vi "why.vi"() -> ()   [LabVIEW 2023]
uses:
  Supporting VIs/Sampling frequency.ctl
  Supporting VIs/Logic states.ctl
  Supporting VIs/Motor states.ctl
  Supporting VIs/Queue names.ctl
  <instrlib>/Arcus Driver 3.0.0/ArcusUsbComm/classes/Controller/_Controller.lvclass
  <instrlib>/Arcus Driver 3.0.0/ArcusUsbComm/common/controls/linear_direction.ctl
  Supporting VIs/Axes indices.ctl
  <vilib>/DAQmx/read.llb/DAQmx Read (Analog 1D DBL NChan 1Samp).vi
  <vilib>/Analysis/baseanly.llb/Vector x A.vi
  <vilib>/Analysis/baseanly.llb/A x Vector.vi
  <vilib>/DAQmx/create/channels.llb/DAQmx Create Channel (AI-Voltage-Basic).vi
  <vilib>/DAQmx/configure/timing.llb/DAQmx Timing (Sample Clock).vi
  <vilib>/DAQmx/miscellaneous.llb/DAQmx Fill In Error Info.vi
  <vilib>/Utility/file.llb/Write Delimited Spreadsheet (string).vi
  <vilib>/Utility/file.llb/Write Delimited Spreadsheet (DBL).vi
  <vilib>/addons/control/pid/pid.llb/PID (DBL).vi
  <vilib>/Analysis/NI_AALBase.lvlib
  <instrlib>/Arcus Driver 3.0.0/ArcusUsbComm/libraries/common.lvlib
  <vilib>/addons/control/pid/NI_PID_pid.lvlib
  <instrlib>/Zaber A Series/Zaber A Series.lvlib
panel:
  out "Steady State COFs":dbl[](array[numeric])
  out "Fixed amplitude Load":dbl(graph)=8.923720573303449
  in  "VISA resource name":refnum<visa-resource-name>
  out "Mean Estimated Friction Coefficient":dbl[](array[numeric])
  in  "Maximum COF Difference":i32=3000
  in  "Number of Previous Points":i32=3000
  out "Torque":dbl(graph)=-1.1532615270996815
  out "Sliding Distance (mm)":i32
  out "Angular Position":dbl
  in  "Initial Position":dbl
  in  "Track Radius (mm)":T1=100 items=["4 mm"=4, "6 mm"=6, "8 mm"=8, "10 mm"=10, "12 mm"=12, "14 mm"=14, "16 mm"=16, "18 mm"=18]
  out "Revolutions Completed":u8(slide) scale=0.0..10.0
  in  "STOP Rotating Motor":bool
  in  "Clockwise":bool
  in  "Number of Revolutions":i32
  out "Progress":dbl(slide) scale=0.0..100.0
  in  "Velocity":dbl
  in  "Units (0: microsteps)":u16(ring) items=["device speed units", "microns per second", "millimeters per second", "inches per second", "degrees per second"]
  in  "Microstep Size (0)":dbl
  in  "Wait [min]":dbl=30.0 format="%.2g"
  in  "Wait ?":bool=TRUE
  in  "Save file name":path=path "C:/Users/Egberts/Desktop/Tribometer/August 2020 Measurements/Tribometer/Late August 2020/test.txt"
  in  "PID gains":T2={"proportional gain (Kc)"=0.02, "integral time (Ti, min)"=0.1, "derivative time (Td, min)"=0.001} {"derivative time (Td, min)" format="%.3f"; "integral time (Ti, min)" format="%.3f"; "proportional gain (Kc)" format="%.3f"}
  in  "output range":cluster{"output high":dbl, "output low":dbl}={"output high"=2.0, "output low"=-2.0} {"output low" format="%.2f"; "output high" format="%.2f"}
  out "x-position":i32
  out "z-position":string
  in  "set zero":bool
  out "Correction loop":i32
  out "received P":i32
  out "Actual Load":dbl
  out "Correction [N]":dbl format="%.2f"
  out "correction [p]":dbl
  out "to PID":i32
  out "dt out (s)":dbl=0.25 format="%.3f"
  in  "Testing Load [N]":dbl=20.0
  in  "Wear cycles":i32=3000
  out "Manual control":bool
  in  "Approach":bool
  in  "DAQmx Device Name":tag="Dev1"
  in  "Out":bool
  in  "In":bool
  in  "Left":bool
  in  "Right":bool
  in  "Up":bool
  out "Estimated friction coefficient":dbl(graph)=-0.11599973982411911
  out "Smooth Force from Torque":dbl(graph)=-1.1532615270996815
  out "Smooth z":dbl(graph)=9.94193201509139
  out "Dequeued Data":dbl[](graph)=[9.378691263157721, 10.717600289594278, 8.438969804942502, 9.318124790458075, 8.681089909963866, 9.970529667476073, 10.834102440336615, 9.183821958337319, 9.334582664259113, 9.226213467034226, 10.238553338370796, 11.173780758664948, 8.690449558950064, 9.261606371512476, 8.790570665988898, 9.887706352746802, 11.038667014275244, 8.916330650848511, 9.104119720861869, 8.923720573303449]
  in  "ABORT":bool
  in  "Down":bool
  out "Aborted":bool
  out "Mean z":dbl[](array[numeric])
  out "Current reading":dbl[](array[numeric])
  in  "Averaging Level":i32=12
  out "Mean Force from Torque":dbl[](array[numeric])
  out "Completed":bool
  out "Testing":bool
  out "Approaching":bool
  in  "TARE":bool
  in  "Sampling frequency (rate)":T1=100 items=["1000 Hz"=1000, " 500 Hz"=500, " 250 Hz"=250, "100 Hz"=100, "50 Hz"=50, "10 Hz"=10, "1 Hz"=1]
  in  "Calibration file":path=path "C:/Users/Egberts/Desktop/ATI Industrial Automation/FT21774.cal"
  # "Counterclockwise"
  # "Originally used to measure \nthe amount of positions needed\nto perform fast approach"
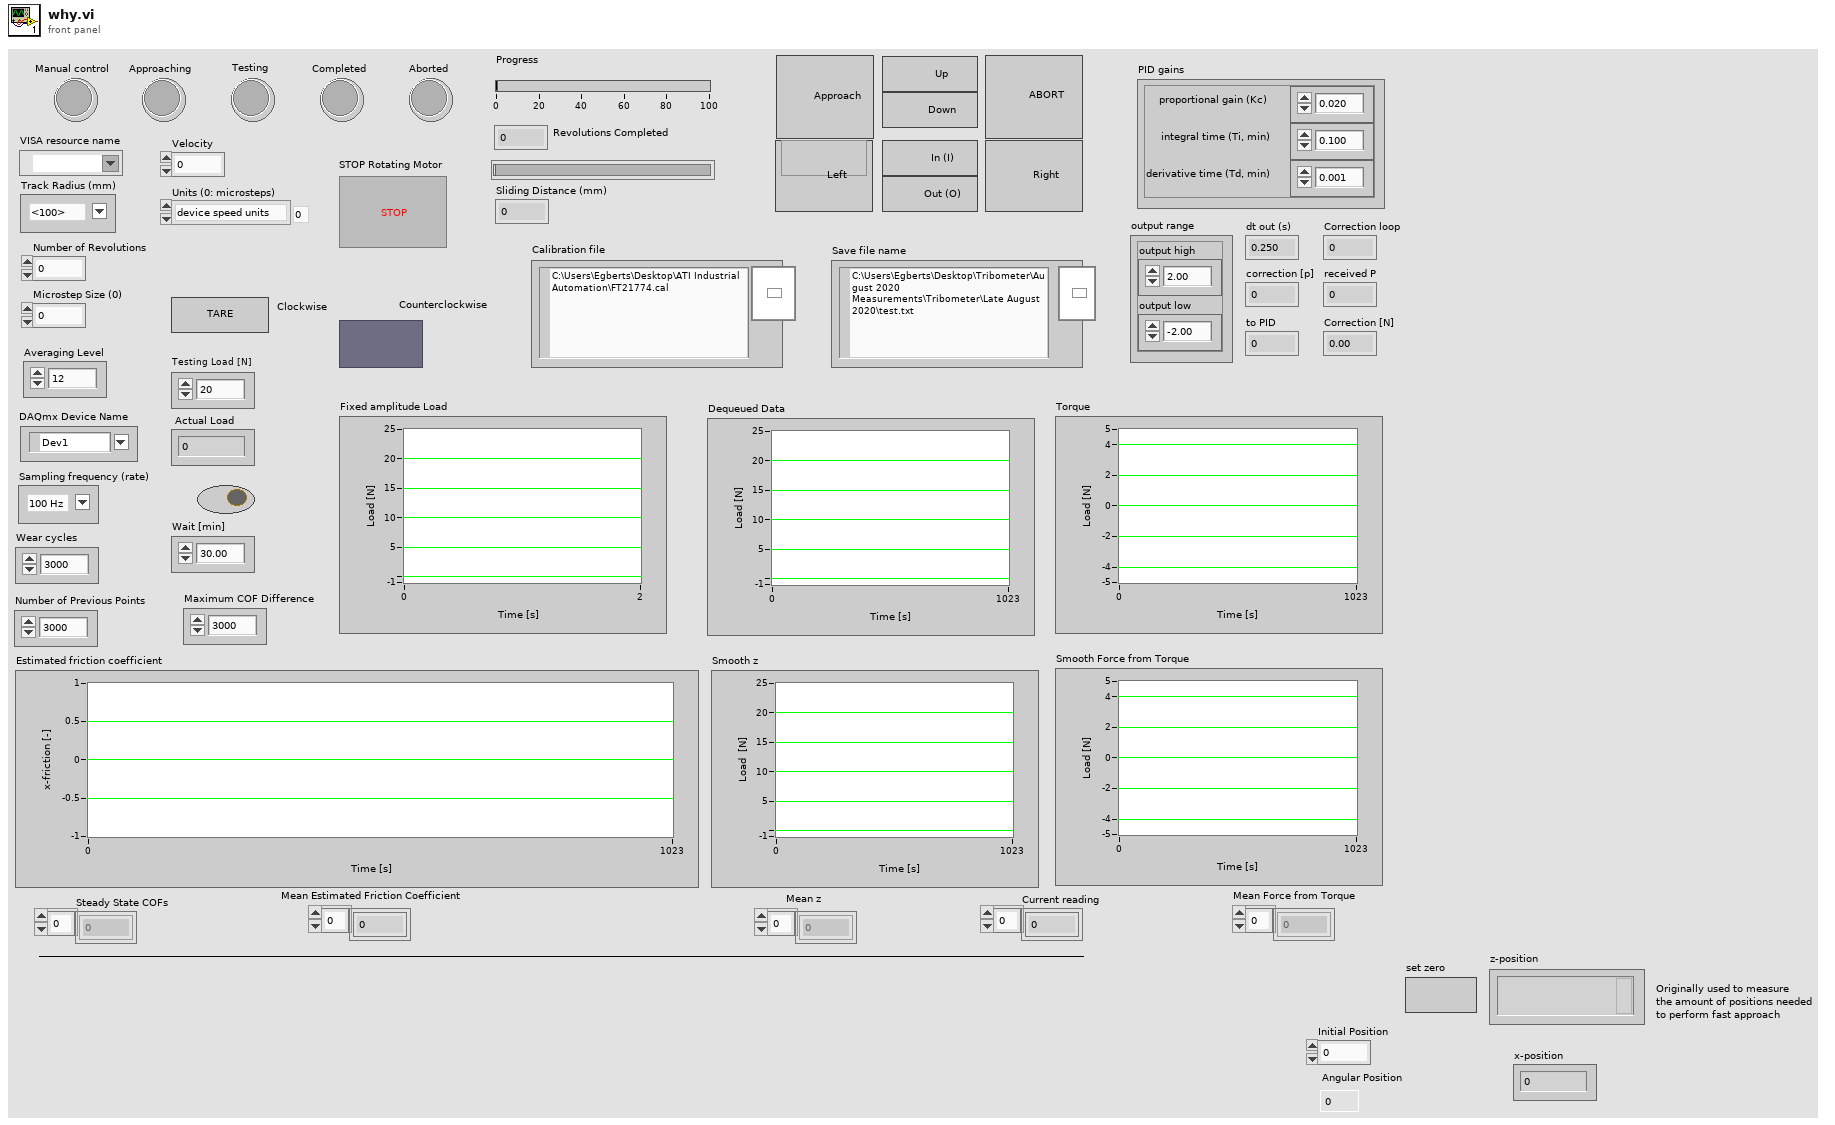
[diagram p1: front panel]
types:
  T1 = typedef "Sampling frequency.ctl" = u16
  T2 = cluster{"proportional gain (Kc)":dbl, "integral time (Ti, min)":dbl, "derivative time (Td, min)":dbl}
  T3 = typedef "Queue names.ctl" = enum16{"Cell queue name", "z-axis ref queue", "x-axis ref queue", "tangent-axis ref queue", "y-axis ref queue", "to PID", "Feedback"}
  T4 = typedef "Motor states.ctl" = enum16{"Initialize", "Manual control", "Approaching", "Testing", "Terminate"}
  T5 = typedef "Logic states.ctl" = enum16{"Initialize", "Process", "Terminate"}
  T6 = enum8{"Enabled", "Disabled", "Disabled and Grayed Out"}
  T7 = cluster{"queue out":refnum<queue>, "error out":errorcluster}
  T8 = cluster{"task out":refnum<k21>, "error out":errorcluster}
  T9 = cluster{"reference (out)":refnum<class "_Controller.lvclass">, "error out":errorcluster}
  T10 = typedef "Axes indices.ctl" = enum16{"y-axis", "x-axis", "z-axis"}
  T11 = cluster{"queue out":refnum<queue>, "queue out":refnum<queue>, "queue out":refnum<queue>}
  T12 = typedef "common.lvlib/linear_direction.ctl" = enum16{"POS (+)", "NEG (-)"}
  T13 = typedef "lveventtype.ctl" = enum32{"Null", "Timeout", "Annotation Menu Selection", "Annotation Menu Selection?", "App Instance Close", "App Instance Close?", "Autoscale Range Change", "Bookmark Info Change", "Cell Edit", "Cell Edit?", "Cursor Grab", "Cursor Grab?", "Cursor Menu Selection", "Cursor Menu Selection?", "Cursor Move", "Cursor Release", "Data Change", "Direction Change", "Display State Change", "Drag Ended", "Drag Enter", "Drag Leave", "Drag Over", "Drag Source Update", "Drag Starting", "Drag Starting?", "Drop", "Exec State Change", "Key Down", "Key Down?", "Key Repeat", "Key Repeat?", "Key Up", "Listbox Double Click", "Menu Activation?", "Menu Selection (App)", "Menu Selection? (App)", "Menu Selection (User)", "Mouse Down", "Mouse Down?", "Mouse Enter", "Mouse Leave", "Mouse Move", "Mouse Up", "Mouse Wheel", "NI Security User Change (App)", "Pane Size", "Panel Close", "Panel Close?", "Panel Resize", "Plot Attribute Change", "Scale Range Change", "Shortcut Menu Activation?", "Shortcut Menu Selection (App)", "Shortcut Menu Selection? (App)", "Shortcut Menu Selection (User)", "Tree Double Click", "Tree Drag", "Tree Drag?", "Tree Drop", "Tree Drop?", "Tree Item Close", "Tree Item Close?", "Tree Item Open", "Tree Item Open?", "User Event", "Value Change"}
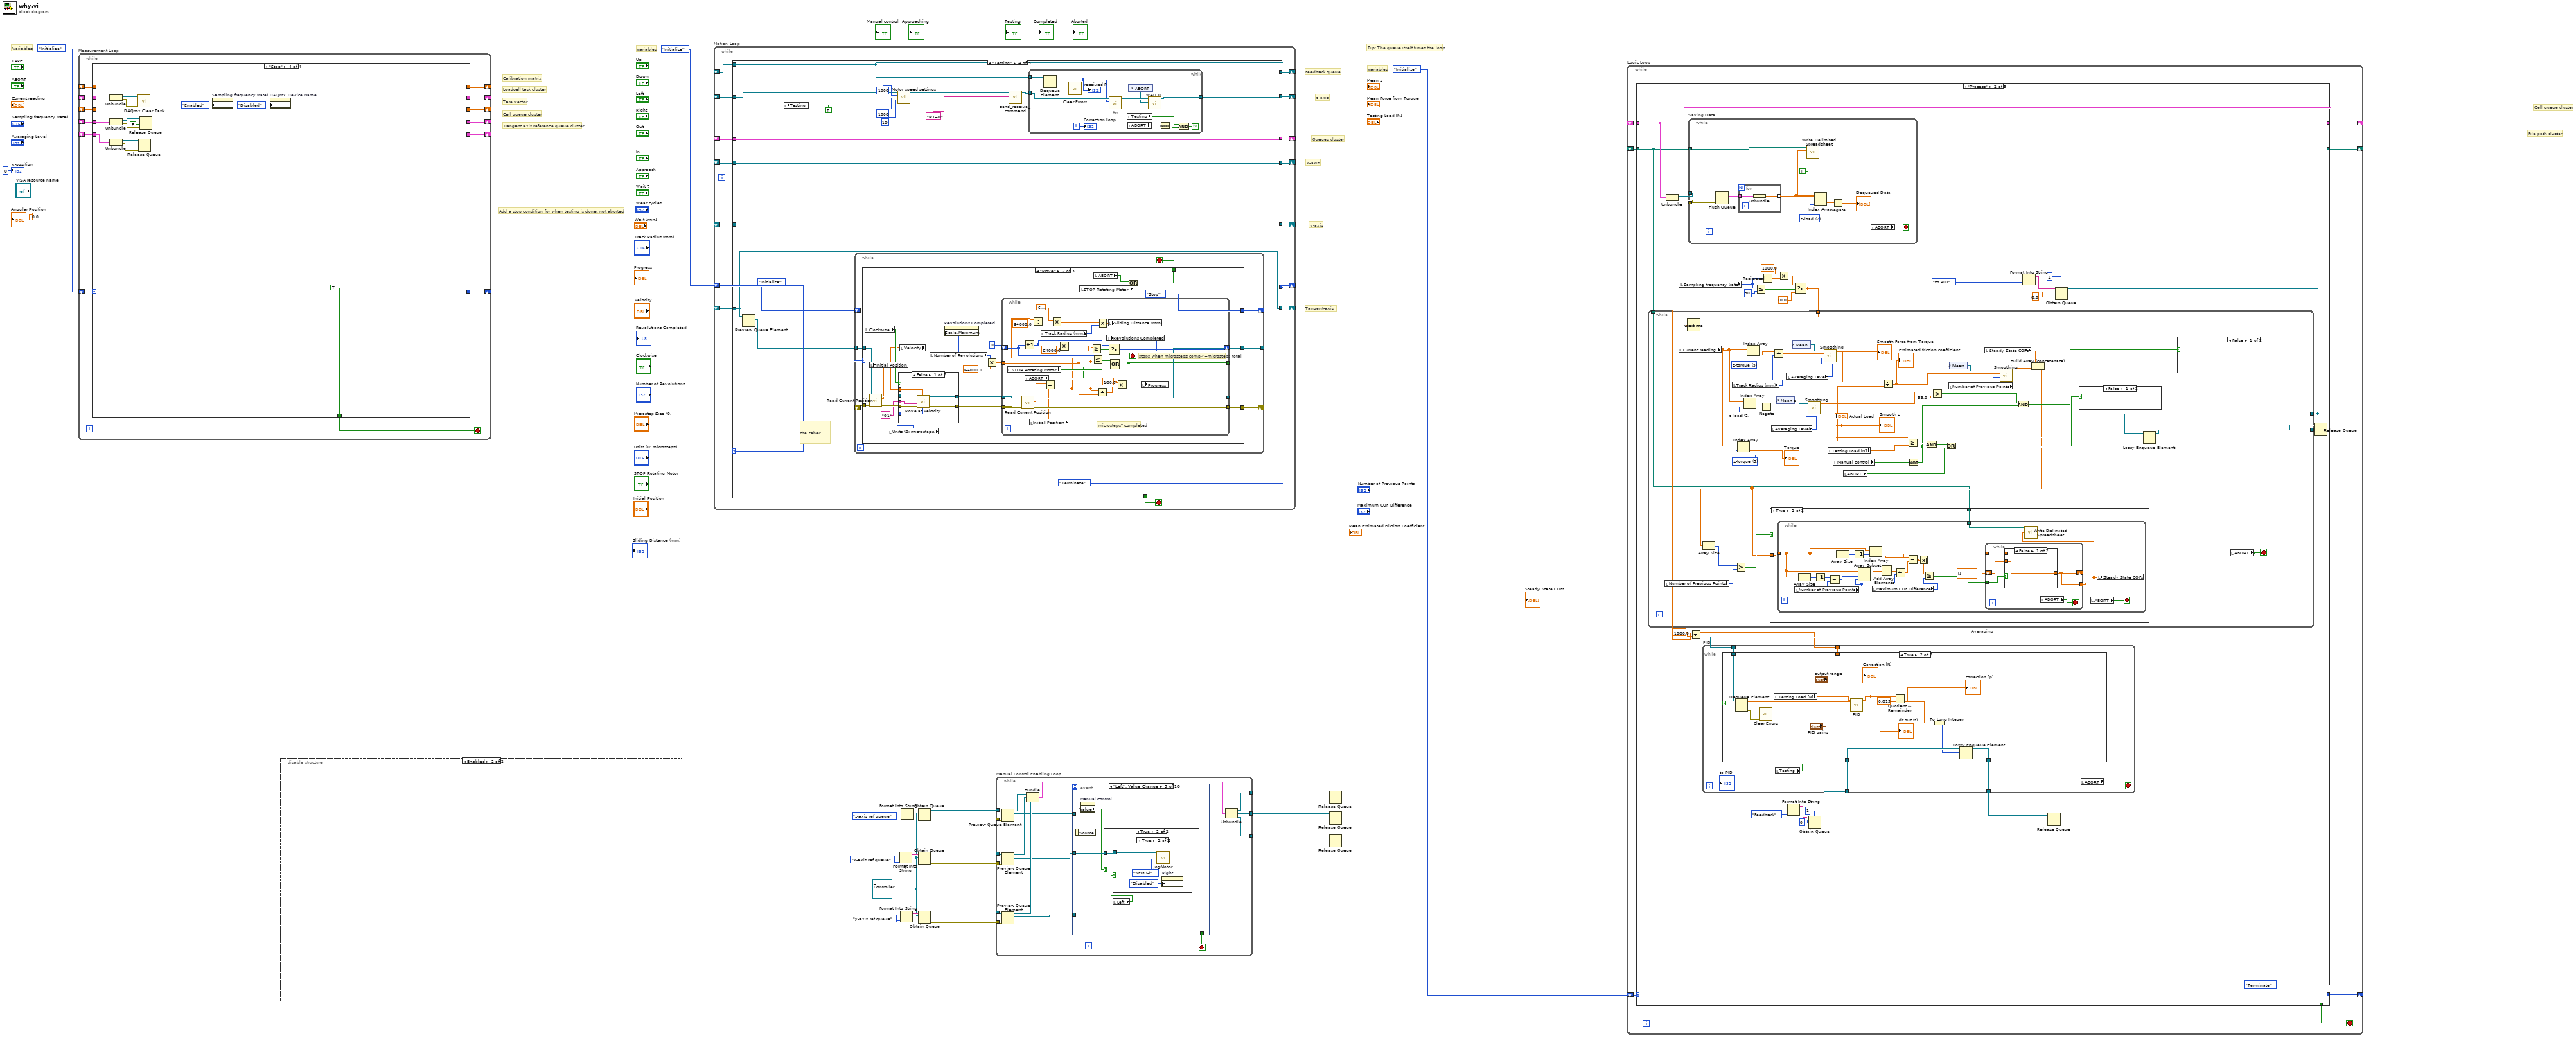
[diagram p0: block diagram]
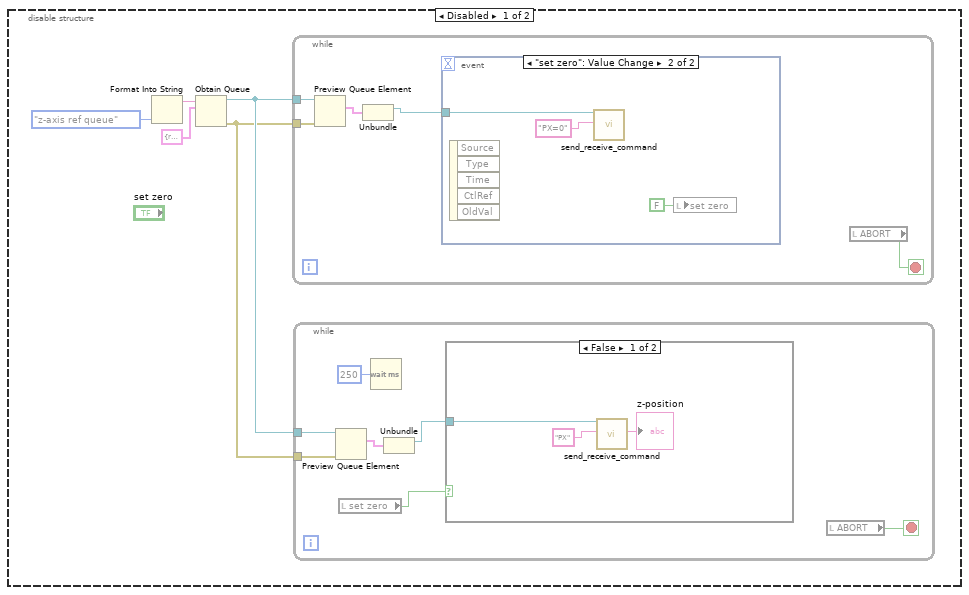
[diagram p2: hidden frame]
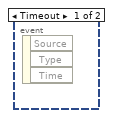
[diagram p4: hidden frame]
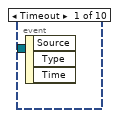
[diagram p5: hidden frame]
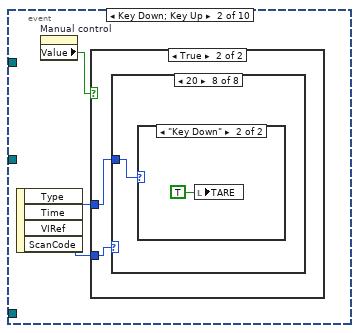
[diagram p6: hidden frame]
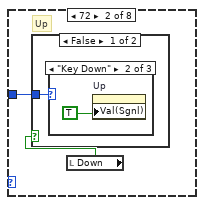
[diagram p9: hidden frame]
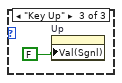
[diagram p11: hidden frame]
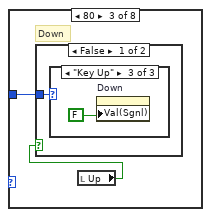
[diagram p13: hidden frame]
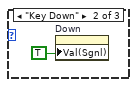
[diagram p15: hidden frame]
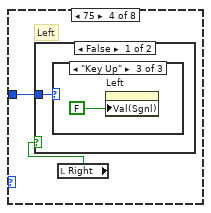
[diagram p17: hidden frame]
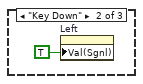
[diagram p19: hidden frame]
diagram:
  w2 = refnum<class "_Controller.lvclass"> refnum ("Controller in")
  # "Tangent-axis"
  # "Feedback queue"
  # "Queues cluster"
  # "Tangent axis reference queue cluster"
  # "Add a stop condition for when testing is done, not aborted"
  # "y-axis"
  # "x-axis"
  # "z-axis"
  # "Variables"
  # "Variables"
  # "File path cluster"
  # "Cell queue cluster"
  # "Tip: The queue itself times the loop"
  # "Variables"
  # "Cell queue cluster"
  # "Loadcell task cluster"
  # "Tare vector"
  # "Calibration matrix"
  n1 = while "Measurement Loop" {
    shift-right: [w33] -> _
    shift-left: enum16{"Initialize", "Tare", "Measure", "Stop"}."Initialize" ("Enum") -> [w34]
    shift-right: [w28] -> _
    shift-left: _ -> [w27]
    shift-right: [w32] -> _
    shift-left: _ -> [w30]
    shift-right: [w31] -> _
    shift-left: _ -> [w29]
    shift-right: [w24] -> _
    shift-left: _ -> [w25]
    shift-right: [w23] -> _
    shift-left: _ -> [w22]
    stop <- w26 stop-if-true
    n2 = case shown="\"Stop\"" w34 {
      tunnel: [w57 w82 w117 _] -> w33
      tunnel: [_ w89 _ _] -> w32
      tunnel: [w61 w81 w119 _] -> w31
      tunnel: w29 -> [_ w81 w119 w185]
      tunnel: w30 -> [_ _ w120 _]
      tunnel: [w60 w88 w118 _] -> w28
      tunnel: w27 -> [_ w88 w118 _]
      tunnel: [_ _ _ TRUE] -> w26
      tunnel: w25 -> [_ w76 w105 w182]
      tunnel: [w52 w76 w106 _] -> w24
      tunnel: [w41 w74 w113 _] -> w23
      tunnel: w22 -> [_ w74 w113 w176]
      frame "Initialize", Default {
        w65 = u16 10123 items=["Continous"=10123, "Finite"=10178, "Hardware Timed"=12522]  # Sample mode
        w72 = "N-M"  # Torque units
        w71 = "N"  # Force units
        n3 = local read "VISA resource name"() -> (w36:refnum<visa-resource-name>)
        n4 = property on="Sampling frequency (rate)" class="Ring (strict)"("DisabledEnum"=T6."Disabled" ("Disabled")) -> ()  [unwired: 2 in, 2 out]
        n5 = call "mxChannelList.vi"("First Channel"=0, "Number of Channels"=6, "DAQmx Device Name"="DAQmx Device Name") -> ("error out"=w67:errorcluster, "Channel List"=w68:string)  [unwired: 1 in]
        n6 = call <instrlib>:"Initialize.vi"("VISA resource name"=w36) -> ("VISA resource name out"=w35:refnum<visa-resource-name>)  [unwired: 9 in, 1 out]
        n7 = call "LoadCalibrationFromFile.vi"("User Torque Units"=w72, "User Force Units"=w71, "Cal File Path"="Calibration file") -> ("Calibration Matrix"=w60:dbl[][])  [unwired: 1 in, 3 out]
        n8 = property on="DAQmx Device Name" class="DAQmxName"("DisabledEnum"=T6."Disabled" ("Disabled")) -> ()  [unwired: 2 in, 2 out]
        n9 = Format Into String(Queue_names."Cell queue name" ("Enum")) -> (resulting string=w39:string)  [unwired: 3 in, 1 out]
        n10 = call-poly <vilib>:"DAQmx Create Virtual Channel.vi"("physical channels"=w68, "error in"=w67) -> ("task out"=w66:refnum<k21>, "error out"=w45:errorcluster)  [unwired: 12 in]
        n11 = local read "Sampling frequency (rate)"() -> (w51:T1)
        n12 = call-poly <vilib>:"DAQmx Timing.vi"("task/channels in"=w66, "sample mode"=w65, "rate"=w51) -> ("task out"=w64:refnum<k21>, "error out"=w63:errorcluster)  [unwired: 11 in]
        n13 = Format Into String(Queue_names."tangent-axis ref queue" ("Enum")) -> (resulting string=w37:string)  [unwired: 3 in, 1 out]
        n14 = call <vilib>:"DAQmx Start Task.vi"("task/channels in"=w64, "error in"=w63) -> ("task out"=w62:refnum<k21>, "error out"=w46:errorcluster)  [unwired: 12 in]
        n15 = Obtain Queue(name (unnamed)=w37, element data type=w35) -> (queue out=w43:refnum<queue>, error out=w42:errorcluster)  [unwired: 3 in, 1 out]
        n16 = Obtain Queue(name (unnamed)=w39, element data type=dbl[] []) -> (queue out=w53:refnum<queue>, error out=w47:errorcluster)  [unwired: 3 in, 1 out]
        n17 = local read "ABORT"() -> (w55:bool)
        n18 = Bundle("queue out"=w53, "error out"=w47) -> (w52:T7)  [unwired: 1 in]
        n19 = Bundle("queue out"=w43, "error out"=w42) -> (w41:T7)  [unwired: 1 in]
        n20 = Bundle("task out"=w62, "error out"=w46) -> (w61:T8)  [unwired: 1 in]
        n21 = Merge Errors(w42, w47, w46, w45) -> (w44:errorcluster)
        n22 = Compound Arithmetic op=OR(w44, w55) -> (w56:bool)
        n23 = Select(t=enum16{"Initialize", "Tare", "Measure", "Stop"}."Stop" ("Enum"), s=w56, f=enum16{"Initialize", "Tare", "Measure", "Stop"}."Tare" ("Enum")) -> (s? t:f=w57:enum16{"Initialize", "Tare", "Measure", "Stop"})
      }
      frame "Tare" {
        n24 = local read "Averaging Level"() -> (w75:i32)
        n25 = for {
          N: w75 -> [_]
          tunnel: w81 -> [w95]
          shift-right: [w97] -> w79
          shift-left: dbl[][] [] -> [w96]
          tunnel: [w94] -> w78
          tunnel: [FALSE] -> w77
          n26 = Unbundle(w95) -> ("task out"=w100:refnum<k21>, "error out"=w99:errorcluster)
          n27 = call-poly <vilib>:"DAQmx Read.vi"("task/channels in"=w100, "error in"=w99) -> ("data"=w98:dbl[], "error out"=w94:errorcluster)  [unwired: 11 in, 1 out]
          n28 = Build Array (concatenate)(w96, w98) -> (w97:dbl[][])
        }
        n29 = local write "TARE"(w77) -> ()
        n30 = Matrix Size(0:w79) -> (1:w90:i32)  [unwired: 1 out]
        n31 = Reciprocal(x=w90) -> (1/x=w91:dbl)
        n32 = Unbundle By Name(w78) -> ("status"=w83:bool)
        n33 = local read "ABORT"() -> (w84:bool)
        n34 = Initialize Array(w91, w90) -> (w92:dbl[])
        n35 = Or(x=w83, y=w84) -> (x .or. y?=w87:bool)
        n36 = call-poly <vilib>:"A x B.vi"("Matrix A"=w79, "Vector V'"=w92) -> ("V' x A"=w89:dbl[])  [unwired: 1 out]
        n37 = Select(t=enum16{"Initialize", "Tare", "Measure", "Stop"}."Stop" ("Enum"), s=w87, f=enum16{"Initialize", "Tare", "Measure", "Stop"}."Measure" ("Enum")) -> (s? t:f=w82:enum16{"Initialize", "Tare", "Measure", "Stop"})
      }
      frame "Measure" {
        n38 = Unbundle(w113) -> ("queue out"=w102:refnum<queue>, "error out"=w101:errorcluster)
        n39 = Unbundle(w105) -> ("queue out"=w104:refnum<queue>, "error out"=w103:errorcluster)
        n40 = Unbundle(w113) -> ("queue out"=w112:refnum<queue>, "error out"=w111:errorcluster)
        n41 = Unbundle(w119) -> ("task out"=w110:refnum<k21>, "error out"=w109:errorcluster)
        n42 = while {
          tunnel: w120 -> [w161]
          tunnel: w118 -> [w153]
          tunnel: [w151] -> w114
          tunnel: w112 -> [w144]
          tunnel: w111 -> [w143]
          tunnel: w110 -> [w142]
          tunnel: w109 -> [w141]
          tunnel: [w140] -> w108
          tunnel: [w139] -> w107
          tunnel: w104 -> [w138]
          tunnel: w103 -> [w137]
          stop <- w156 stop-if-true
          w158 = u16 2 items=["x-load", "y-load", "z-load", "x-torque", "y-torque", "z-torque"]
          n43 = Get Queue Status(queue=w144, error in (no error)=w143) -> (# elements in queue=w148:i32)  [unwired: 1 in, 7 out]
          n44 = local read "Testing"() -> (w147:bool)
          n45 = call-poly <vilib>:"DAQmx Read.vi"("task/channels in"=w142, "error in"=w141) -> ("data"=w154:dbl[], "error out"=w152:errorcluster)  [unwired: 11 in, 1 out]
          n46 = Not Equal To 0?(x=w148) -> (x != 0?=w146:bool)
          n47 = And(x=w146, y=w147) -> (x .and. y?=w145:bool)
          n48 = Subtract(x=w154, y=w161) -> (x-y=w160:dbl[])
          n49 = call-poly <vilib>:"A x B.vi"("Vector"=w160, "A"=w153) -> ("A x Vector"=w149:dbl[])  [unwired: 1 out]
          n50 = case shown="True" w145 {
            tunnel: [FALSE ("status") w173] -> w150
            tunnel: w149 -> [_ w172]
            tunnel: w138 -> [w163 w170]
            tunnel: w137 -> [w162 w169]
            tunnel: [w163 w168] -> w140
            tunnel: [w162 w167] -> w139
            frame False {
            }
            frame True {
              n51 = local read "Angular Position"() -> (w165:dbl)
              n52 = To Long Integer(number=w165) -> (32bit integer=w166:i32)
              n53 = Build Array (concatenate)(w172, w166) -> (w171:dbl[])
              n54 = Enqueue Element(queue=w170, element=w171, error in (no error)=w169) -> (queue out=w168:refnum<queue>, error out=w167:errorcluster)  [unwired: 1 in, 1 out]
              n55 = Unbundle By Name(w167) -> ("status"=w173:bool)
            }
          }
          n56 = local write "Current reading"(w149) -> ()
          n57 = Index Array(array=w149, index=w158) -> (element=w159:dbl)
          n58 = Negate(x=w159) -> (-x=→"Fixed amplitude Load":dbl)
          n59 = local read "TARE"() -> (w151:bool)
          n60 = Unbundle By Name(w152) -> ("status"=w155:bool)
          n61 = local read "ABORT"() -> (w157:bool)
          n62 = Compound Arithmetic op=OR(w150, w151, w157, w155) -> (w156:bool)
        }
        n63 = while {
          tunnel: w102 -> [w122]
          tunnel: w101 -> [w121]
          stop <- w124 stop-if-true
          n64 = local read "Testing"() -> (w128:bool)
          n65 = Get Queue Status(queue=w122, error in (no error)=w121) -> (queue out=w126:refnum<queue>, # elements in queue=w130:i32)  [unwired: 1 in, 6 out]
          n66 = Not Equal To 0?(x=w130) -> (x != 0?=w129:bool)
          n67 = And(x=w129, y=w128) -> (x .and. y?=w127:bool)
          n68 = case shown="True" w127 {
            tunnel: w126 -> [_ w134]
            frame False {
            }
            frame True {
              n69 = Preview Queue Element(queue=w134) -> (element=w133:refnum<visa-resource-name>)  [unwired: 2 in, 3 out]
              n70 = call <instrlib>:"Read Current Position.vi"("Device and Axis"="PX", "VISA resource name"=w133) -> ("VISA resource name out"=w131:refnum<visa-resource-name>)  [unwired: 7 in, 2 out]
              n71 = Decimal String To Number(string=w131) -> (number=w135:i32)  [unwired: 2 in, 1 out]
              n72 = local write "Angular Position"(w135) -> ()
            }
          }
          n73 = local read "ABORT"() -> (w125:bool)
          n74 = local read "TARE"() -> (w123:bool)
          n75 = Or(x=w125, y=w123) -> (x .or. y?=w124:bool)
        }
        n76 = Select(t=enum16{"Initialize", "Tare", "Measure", "Stop"}."Tare" ("Enum"), s=w114, f=enum16{"Initialize", "Tare", "Measure", "Stop"}."Stop" ("Enum")) -> (s? t:f=w117:enum16{"Initialize", "Tare", "Measure", "Stop"})
        n77 = Bundle("queue out"=w108, "error out"=w107) -> (w106:T7)  [unwired: 1 in]
      }
      frame "Stop" {
        n78 = Unbundle(w185) -> ("task out"=w184:refnum<k21>, "error out"=w183:errorcluster)
        n79 = Unbundle(w182) -> ("queue out"=w181:refnum<queue>, "error out"=w180:errorcluster)
        n80 = Unbundle(w176) -> ("queue out"=w175:refnum<queue>, "error out"=w174:errorcluster)
        n81 = call <vilib>:"DAQmx Clear Task.vi"("task in"=w184, "error in"=w183) -> ()  [unwired: 13 in, 1 out]
        n82 = Release Queue(queue=w175, error in (no error)=w174) -> ()  [unwired: 1 in, 3 out]
        n83 = Release Queue(queue=w181, force destroy? (F)=FALSE, error in (no error)=w180) -> ()  [unwired: 3 out]
        n84 = property on="Sampling frequency (rate)" class="Ring (strict)"("DisabledEnum"=T6."Enabled" ("Disabled")) -> ()  [unwired: 2 in, 2 out]
        n85 = property on="DAQmx Device Name" class="DAQmxName"("DisabledEnum"=T6."Disabled" ("Disabled")) -> ()  [unwired: 2 in, 2 out]
      }
    }
  }
  n86 = disable-structure shown="Enabled" {
    frame Disabled {
      n87 = Format Into String(Queue_names."z-axis ref queue" ("Enum")) -> (resulting string=w190:string)  [unwired: 3 in, 1 out]
      n88 = Obtain Queue(name (unnamed)=w190, element data type=T9 {"reference (out)"=refnum, "error out"={"status"=FALSE, "code"=0, "source"=""}} ("output cluster")) -> (queue out=w188:refnum<queue>, error out=w187:errorcluster)  [unwired: 3 in, 1 out]
      n89 = while {
        tunnel: w188 -> [w206]
        tunnel: w187 -> [w205]
        stop <- w202 stop-if-true
        n90 = Preview Queue Element(queue=w206, error in (no error)=w205) -> (element=w204:T9)  [unwired: 1 in, 3 out]
        n91 = Unbundle(w204) -> ("reference (out)"=w203:refnum<class "_Controller.lvclass">)  [unwired: 1 out]
        n92 = event shown="[1] \"set zero\": Value Change" {
          selector: _ -> [_ _]
          dyn-events: _ -> [_ _]
          timeout: _ -> [_ _]
          tunnel: w203 -> [_ w209]
          event Timeout {
            n93 = event-data() -> ()  [unwired: 1 in, 3 out]
          }
          event "set zero": Value Change {
            n94 = event-data() -> ()  [unwired: 1 in, 5 out]
            n95 = call <instrlib>:"send_receive_command.vi"("reference (in)"=w209, "ASCII Command (in)"="PX=0") -> ()  [unwired: 13 in, 5 out]
            n96 = local write "set zero"(FALSE ("set zero")) -> ()
          }
        }
        n97 = local read "ABORT"() -> (w202:bool)
      }
      n98 = while {
        tunnel: w188 -> [w195]
        tunnel: w187 -> [w194]
        stop <- w197 stop-if-true
        n99 = Preview Queue Element(queue=w195, error in (no error)=w194) -> (element=w196:T9)  [unwired: 1 in, 3 out]
        n100 = local read "set zero"() -> (w192:bool)
        n101 = Wait (ms)(milliseconds to wait=u32 250) -> ()  [unwired: 1 out]
        n102 = Unbundle(w196) -> ("reference (out)"=w193:refnum<class "_Controller.lvclass">)  [unwired: 1 out]
        n103 = case shown="False" w192 {
          tunnel: w193 -> [w200 _]
          frame False {
            n104 = call <instrlib>:"send_receive_command.vi"("reference (in)"=w200, "ASCII Command (in)"="PX") -> ("response (out)"=→"z-position":string)  [unwired: 13 in, 4 out]
          }
          frame True {
          }
        }
        n105 = local read "ABORT"() -> (w197:bool)
      }
    }
    frame Enabled {
    }
  }
  n106 = while "Motion Loop" {
    shift-right: [w223] -> _
    shift-left: Motor_states."Initialize" -> [w224]
    shift-right: [w215] -> _
    shift-left: _ -> [w222]
    shift-right: [w214] -> _
    shift-left: _ -> [w212]
    shift-right: [w213] -> _
    shift-left: _ -> [w221]
    shift-right: [w219] -> _
    shift-left: _ -> [w218]
    shift-right: [w217] -> _
    shift-left: _ -> [w216]
    shift-right: [w211] -> _
    shift-left: _ -> [w210]
    stop <- w220 stop-if-true
    n107 = case shown="\"Testing\"" w224 {
      tunnel: [Motor_states."Manual control" w294 w316 Motor_states."Terminate" _] -> w223
      tunnel: w222 -> [_ w279 w307 w365 w478]
      tunnel: w221 -> [_ w275 w309 w363 w476]
      tunnel: [_ _ _ _ w484] -> w220
      tunnel: [w243 w281 w312 w370 _] -> w219
      tunnel: w218 -> [_ w281 w312 w370 w483]
      tunnel: [w238 w280 w311 w369 _] -> w217
      tunnel: w216 -> [_ w280 w311 w369 w479]
      tunnel: [w237 w278 w310 w364 _] -> w215
      tunnel: [w236 w276 w304 w362 _] -> w214
      tunnel: [w235 w274 w309 w363 _] -> w213
      tunnel: w212 -> [_ w277 w305 w362 w477]
      tunnel: [w228 w273 w303 w359 _] -> w211
      tunnel: w210 -> [_ w273 w303 w359 _]
      frame "Initialize" {
        w225 = TRUE
        w234 = FALSE ("Approach")
        n108 = local write "Testing"(w234) -> ()
        n109 = local write "Aborted"(w234) -> ()
        n110 = local write "Approach"(w234) -> ()
        n111 = local write "Approaching"(w234) -> ()
        n112 = local write "Completed"(w234) -> ()
        n113 = local write "Progress"(0 ("Test Progress")) -> ()
        n114 = local read "VISA resource name"() -> (w230:refnum<visa-resource-name>)
        n115 = call <instrlib>:"initialize.vi"("device_index (in) [0=def]"=Axes_indices."x-axis", "clear_buffer? (T)"=w225) -> ("reference (out)"=w267:refnum<class "_Controller.lvclass">)  [unwired: 16 in, 1 out]
        n116 = call <instrlib>:"initialize.vi"("device_index (in) [0=def]"=Axes_indices."y-axis", "clear_buffer? (T)"=w225) -> ("reference (out)"=w266:refnum<class "_Controller.lvclass">)  [unwired: 16 in, 1 out]
        n117 = call <instrlib>:"initialize.vi"("device_index (in) [0=def]"=Axes_indices."z-axis", "clear_buffer? (T)"=w225) -> ("reference (out)"=w268:refnum<class "_Controller.lvclass">)  [unwired: 16 in, 1 out]
        n118 = call <instrlib>:"send_receive_command.vi"("reference (in)"=w267, "ASCII Command (in)"="SR0=0") -> ("reference (out)"=w261:refnum<class "_Controller.lvclass">)  [unwired: 13 in, 4 out]
        n119 = call <instrlib>:"send_receive_command.vi"("reference (in)"=w266, "ASCII Command (in)"="SR0=0") -> ("reference (out)"=w262:refnum<class "_Controller.lvclass">)  [unwired: 13 in, 4 out]
        n120 = call <instrlib>:"send_receive_command.vi"("reference (in)"=w268, "ASCII Command (in)"="SR0=0") -> ("reference (out)"=w260:refnum<class "_Controller.lvclass">)  [unwired: 13 in, 4 out]
        n121 = call <instrlib>:"Initialize.vi"("VISA resource name"=w230) -> ("VISA resource name out"=w226:refnum<visa-resource-name>)  [unwired: 9 in, 1 out]
        n122 = call <instrlib>:"send_receive_command.vi"("reference (in)"=w261, "ASCII Command (in)"="INC") -> ("reference (out)"=w236:refnum<class "_Controller.lvclass">)  [unwired: 13 in, 4 out]
        n123 = call <instrlib>:"send_receive_command.vi"("reference (in)"=w262, "ASCII Command (in)"="INC") -> ("reference (out)"=w235:refnum<class "_Controller.lvclass">)  [unwired: 13 in, 4 out]
        n124 = call <instrlib>:"send_receive_command.vi"("reference (in)"=w260, "ASCII Command (in)"="INC") -> ("reference (out)"=w237:refnum<class "_Controller.lvclass">)  [unwired: 13 in, 4 out]
        n125 = Format Into String(Queue_names."tangent-axis ref queue" ("Enum")) -> (resulting string=w231:string)  [unwired: 3 in, 1 out]
        n126 = Obtain Queue(name (unnamed)=w231, element data type=w226) -> (queue out=w229:refnum<queue>, error out=w227:errorcluster)  [unwired: 3 in, 1 out]
        n127 = Enqueue Element(queue=w229, element=w226, error in (no error)=w227) -> (queue out=w228:refnum<queue>)  [unwired: 1 in, 2 out]
        n128 = Format Into String(Queue_names."Feedback" ("Enum")) -> (resulting string=w242:string)  [unwired: 3 in, 1 out]
        n129 = Format Into String(Queue_names."y-axis ref queue" ("Enum")) -> (resulting string=w250:string)  [unwired: 3 in, 1 out]
        n130 = Format Into String(Queue_names."x-axis ref queue" ("Enum")) -> (resulting string=w251:string)  [unwired: 3 in, 1 out]
        n131 = Format Into String(Queue_names."z-axis ref queue" ("Enum")) -> (resulting string=w252:string)  [unwired: 3 in, 1 out]
        n132 = Obtain Queue(max queue size (-1, unlimited)=1, name (unnamed)=w242, element data type=0) -> (queue out=w238:refnum<queue>)  [unwired: 2 in, 2 out]
        n133 = Obtain Queue(name (unnamed)=w250, element data type=w235) -> (queue out=w257:refnum<queue>, error out=w256:errorcluster)  [unwired: 3 in, 1 out]
        n134 = Obtain Queue(name (unnamed)=w251, element data type=w236) -> (queue out=w258:refnum<queue>)  [unwired: 3 in, 2 out]
        n135 = Obtain Queue(name (unnamed)=w252, element data type=w237) -> (queue out=w259:refnum<queue>)  [unwired: 3 in, 2 out]
        n136 = Enqueue Element(queue=w258, element=w236) -> (queue out=w245:refnum<queue>)  [unwired: 2 in, 2 out]
        n137 = Enqueue Element(queue=w257, element=w235, error in (no error)=w256) -> (queue out=w244:refnum<queue>)  [unwired: 1 in, 2 out]
        n138 = Enqueue Element(queue=w259, element=w237) -> (queue out=w246:refnum<queue>)  [unwired: 2 in, 2 out]
        n139 = Bundle("queue out"=w246, "queue out"=w245, "queue out"=w244) -> (w243:T11)  [unwired: 1 in]
      }
      frame "Manual control" {
        n140 = while {
          tunnel: [w300] -> w283
          stop <- w299 stop-if-true
          n141 = Wait Until Next ms Multiple(millisecond multiple=u32 150) -> ()  [unwired: 1 out]
          n142 = local read "Approach"() -> (w301:bool)
          n143 = local read "ABORT"() -> (w300:bool)
          n144 = Or(x=w301, y=w300) -> (x .or. y?=w299:bool)
        }
        n145 = local write "Manual control"(TRUE ("Manual control")) -> ()
        n146 = call "Motor speed settings.vi"("reference (in)"=w275, "HSPD"=13000 ("High Speed"), "LSPD"=100 ("Low Speed"), "ACC"=250 ("Acceleration Time")) -> ("reference (out)"=w274:refnum<class "_Controller.lvclass">)  [unwired: 10 in, 1 out]
        n147 = call "Motor speed settings.vi"("reference (in)"=w279, "HSPD"=13000 ("High Speed"), "LSPD"=100 ("Low Speed"), "ACC"=250 ("Acceleration Time")) -> ("reference (out)"=w278:refnum<class "_Controller.lvclass">)  [unwired: 10 in, 1 out]
        n148 = call "Motor speed settings.vi"("reference (in)"=w277, "HSPD"=13000 ("High Speed"), "LSPD"=100 ("Low Speed"), "ACC"=250 ("Acceleration Time")) -> ("reference (out)"=w276:refnum<class "_Controller.lvclass">)  [unwired: 10 in, 1 out]
        n149 = case shown="False" w283 {
          tunnel: [FALSE TRUE] -> w282
          frame False {
          }
          frame True {
          }
        }
        n150 = local write "Manual control"(w282) -> ()
        n151 = Select(t=Motor_states."Terminate", s=w283, f=Motor_states."Approaching") -> (s? t:f=w294:T4)
      }
      frame "Approaching" {
        n152 = flat-sequence {
          tunnel: w307 -> [w320]
          tunnel: [w319] -> w306
          tunnel: [w329] -> w308
          tunnel: w306 -> [w328]
          tunnel: w305 -> [w327]
          tunnel: [w326] -> w304
          frame #0 {
            n153 = local read "Wait ?"() -> (w321:bool)
            n154 = case shown="True" w321 {
              tunnel: w320 -> [w322 w323]
              tunnel: [w322 w323] -> w319
              frame False {
              }
              frame True {
                n155 = control-ref of="ABORT"() -> (w325:refnum<vi>)
                n156 = control-ref of="Wait [min]"() -> (w324:refnum<vi>)
                n157 = call "PASSIVATE.vi"("reference"=w324, "Boolean in"=w325) -> ()  [unwired: 1 in]
              }
            }
          }
          frame #1 {
            n158 = call "Motor speed settings.vi"("reference (in)"=w328, "HSPD"=22000 ("High Speed"), "LSPD"=1000 ("Low Speed"), "ACC"=500 ("Acceleration Time")) -> ("reference (out)"=w338:refnum<class "_Controller.lvclass">)  [unwired: 10 in, 1 out]
            n159 = call "Motor speed settings.vi"("reference (in)"=w327, "HSPD"=1000, "LSPD"=1000, "ACC"=10) -> ("reference (out)"=w345:refnum<class "_Controller.lvclass">)  [unwired: 10 in, 1 out]
            n160 = local read "Track Radius (mm)"() -> (w347:T1)
            n161 = control-ref of="ABORT"() -> (w339:refnum<vi>)
            n162 = call "Xn.vi"("Position"=55000, "_Controller in"=w338) -> ("_Controller out"=w340:refnum<class "_Controller.lvclass">)  [unwired: 8 in, 1 out]
            n163 = call "WAIT 0.vi"("reference"=w339, "_Controller in"=w340) -> ("_Controller out"=w337:refnum<class "_Controller.lvclass">)  [unwired: 7 in, 2 out]
            n164 = control-ref of="ABORT"() -> (w349:refnum<vi>)
            n165 = Multiply(x=w347, y=800) -> (x*y=w348:i32)
            n166 = call "Xn.vi"("Position"=w348, "_Controller in"=w345) -> ("_Controller out"=w346:refnum<class "_Controller.lvclass">)  [unwired: 8 in, 1 out]
            n167 = call "Motor speed settings.vi"("reference (in)"=w337, "HSPD"=100 ("High Speed"), "LSPD"=100 ("Low Speed"), "ACC"=10 ("Acceleration Time")) -> ("reference (out)"=w329:refnum<class "_Controller.lvclass">)  [unwired: 10 in, 1 out]
            n168 = call "WAIT 0.vi"("reference"=w349, "_Controller in"=w346) -> ("_Controller out"=w326:refnum<class "_Controller.lvclass">)  [unwired: 7 in, 2 out]
          }
        }
        n169 = local write "Approaching"(TRUE ("Approaching")) -> ()
        n170 = while {
          tunnel: [w352] -> w310
          tunnel: [w355] -> w315
          tunnel: [w354] -> w313
          tunnel: w308 -> [w350]
          stop <- w354 continue-if-true
          n171 = local read "Approaching"() -> (w358:bool)
          n172 = local read "ABORT"() -> (w355:bool)
          n173 = control-ref of="ABORT"() -> (w351:refnum<vi>)
          n174 = call "Xn.vi"("Position"=15, "_Controller in"=w350) -> ("_Controller out"=w353:refnum<class "_Controller.lvclass">)  [unwired: 8 in, 1 out]
          n175 = Not(x=w355) -> (.not. x?=w356:bool)
          n176 = And(x=w358, y=w356) -> (x .and. y?=w354:bool)
          n177 = call "WAIT 0.vi"("reference"=w351, "_Controller in"=w353) -> ("_Controller out"=w352:refnum<class "_Controller.lvclass">)  [unwired: 7 in, 2 out]
        }
        n178 = Select(t=Motor_states."Terminate", s=w315, f=Motor_states."Testing") -> (s? t:f=w316:T4)
        n179 = local write "Approaching"(w313) -> ()
      }
      frame "Testing" {
        # "the zaber"
        n180 = Preview Queue Element(queue=w359) -> (element=w360:refnum<visa-resource-name>)  [unwired: 2 in, 3 out]
        n181 = local write "Testing"(TRUE ("Testing")) -> ()
        n182 = while {
          shift-right: [w381] -> _
          shift-left: enum16{"Initialize", "Move", "Stop"}."Initialize" -> [w382]
          shift-right: [w380] -> _
          shift-left: _ -> [w379]
          tunnel: w360 -> [w377]
          tunnel: [w376] -> _
          stop <- w378 stop-if-true
          n183 = case shown="\"Move\"" w382 {
            tunnel: [enum16{"Initialize", "Move", "Stop"}."Move" enum16{"Initialize", "Move", "Stop"}."Stop" _] -> w381
            tunnel: [w388 w398 _] -> w380
            tunnel: w379 -> [_ w399 w456]
            tunnel: [w385 w394 TRUE] -> w378
            tunnel: w377 -> [w383 w393 w454]
            tunnel: [w384 w392 _] -> w376
            frame "Initialize", Default {
              n184 = call <instrlib>:"Initialize.vi"("VISA resource name"=w383) -> ("error out"=w388:errorcluster, "VISA resource name out"=w384:refnum<visa-resource-name>)  [unwired: 9 in]
              n185 = local read "STOP Rotating Motor"() -> (w386:bool)
              n186 = local read "ABORT"() -> (w387:bool)
              n187 = Or(x=w387, y=w386) -> (x .or. y?=w385:bool)
            }
            frame "Move" {
              n188 = local read "Clockwise"() -> (w410:bool)
              n189 = call <instrlib>:"Read Current Position.vi"("error in (no error)"=w399, "VISA resource name"=w393) -> ("error out"=w404:errorcluster, "Position"=w403:dbl, "VISA resource name out"=w405:refnum<visa-resource-name>)  [unwired: 7 in]
              n190 = local write "Initial Position"(w403) -> ()
              n191 = local read "Units (0: microsteps)"() -> (w408:u16)
              n192 = local read "Velocity"() -> (w409:dbl)
              n193 = case shown="False" w410 {
                tunnel: w409 -> [w442 w453]
                tunnel: w408 -> [w439 w451]
                tunnel: w404 -> [w441 w449]
                tunnel: "01" ("Device and Axis") -> [w438 w448]
                tunnel: w405 -> [w444 w447]
                tunnel: [w440 w446] -> w407
                tunnel: [w443 w445] -> w406
                frame False {
                  n194 = call <instrlib>:"Move at Velocity.vi"("Units (0: device speed units)"=w439, "Velocity"=w442, "error in (no error)"=w441, "Device and Axis"=w438, "VISA resource name"=w444) -> ("error out"=w440:errorcluster, "VISA resource name out"=w443:refnum<visa-resource-name>)  [unwired: 5 in]
                }
                frame True {
                  n195 = Multiply(x=-1.0, y=w453) -> (x*y=w450:dbl)
                  n196 = call <instrlib>:"Move at Velocity.vi"("Units (0: device speed units)"=w451, "Velocity"=w450, "error in (no error)"=w449, "Device and Axis"=w448, "VISA resource name"=w447) -> ("error out"=w446:errorcluster, "VISA resource name out"=w445:refnum<visa-resource-name>)  [unwired: 5 in]
                }
              }
              n197 = local read "Number of Revolutions"() -> (w397:i32)
              n198 = property on="Revolutions Completed" class="Slide (strict)"("Scale.Maximum"=w397) -> ()  [unwired: 2 in, 2 out]
              n199 = Multiply(x=w397, y=64000.0) -> (x*y=w402:dbl)
              n200 = while {
                tunnel: [w436] -> w392
                tunnel: [w435] -> w398
                tunnel: w407 -> [w434]
                tunnel: w406 -> [w433]
                tunnel: w402 -> [w425]
                tunnel: [w432] -> _
                shift-right: [w419] -> _
                shift-left: 0 -> [w420]
                stop <- w432 stop-if-true
                # "stops when microsteps comp>=microsteps total"
                # "microsteps? completed"
                n201 = local read "STOP Rotating Motor"() -> (w437:bool)
                n202 = call <instrlib>:"Read Current Position.vi"("error in (no error)"=w434, "VISA resource name"=w433) -> ("error out"=w435:errorcluster, "Position"=w430:dbl, "VISA resource name out"=w436:refnum<visa-resource-name>)  [unwired: 7 in]
                n203 = Increment(x=w420) -> (x+1=w423:i32)
                n204 = local read "ABORT"() -> (w418:bool)
                n205 = local read "Initial Position"() -> (w429:dbl)
                n206 = local read "Track Radius (mm)"() -> (w412:T1)
                n207 = Subtract(x=w430, y=w429) -> (x-y=w416:dbl)
                n208 = Divide(x=w416, y=64000.0) -> (x/y=w414:dbl)
                n209 = Multiply(x=6.283185307179586, y=w414) -> (x*y=w413:dbl)
                n210 = Multiply(x=w423, y=64000.0) -> (x*y=w422:dbl)
                n211 = Greater Or Equal?(x=w416, y=w422) -> (x >= y?=w421:bool)
                n212 = Less Or Equal?(x=w425, y=w416) -> (x <= y?=w431:bool)
                n213 = Divide(x=w416, y=w425) -> (x/y=w428:dbl)
                n214 = Multiply(x=w413, y=w412) -> (x*y=w411:dbl)
                n215 = local write "Sliding Distance (mm)"(w411) -> ()
                n216 = Select(t=w423, s=w421, f=w420) -> (s? t:f=w419:i32)
                n217 = local write "Revolutions Completed"(w419) -> ()
                n218 = Compound Arithmetic op=OR(w431, w437, w418) -> (w432:bool)
                n219 = Multiply(x=100.0, y=w428) -> (x*y=w427:dbl)
                n220 = local write "Progress"(w427) -> ()
              }
              n221 = local read "STOP Rotating Motor"() -> (w396:bool)
              n222 = local read "ABORT"() -> (w395:bool)
              n223 = Or(x=w395, y=w396) -> (x .or. y?=w394:bool)
            }
            frame "Stop" {
              n224 = call <instrlib>:"Stop.vi"("error in (no error)"=w456, "VISA resource name"=w454) -> ("error out"=w457:errorcluster, "VISA resource name out"=w458:refnum<visa-resource-name>)  [unwired: 8 in]
              n225 = call <instrlib>:"Close.vi"("error in (no error)"=w457, "VISA resource name"=w458) -> ()  [unwired: 9 in, 1 out]
            }
          }
        }
        n226 = call "Motor speed settings.vi"("reference (in)"=w365, "HSPD"=1000, "LSPD"=1000, "ACC"=10) -> ("reference (out)"=w367:refnum<class "_Controller.lvclass">)  [unwired: 10 in, 1 out]
        n227 = call <instrlib>:"send_receive_command.vi"("reference (in)"=w367, "ASCII Command (in)"="PX=0") -> ("reference (out)"=w366:refnum<class "_Controller.lvclass">)  [unwired: 13 in, 4 out]
        n228 = while {
          tunnel: w366 -> [w470]
          tunnel: [w460] -> w364
          tunnel: w369 -> [w461]
          i -> [w468]
          stop <- w464 continue-if-true
          n229 = Dequeue Element(queue=w461) -> (element=w462:i32, error out=w463:errorcluster)  [unwired: 2 in, 2 out]
          "received P" <- w462
          n230 = call <vilib>:"Clear Errors.vi"("error in (no error)"=w463) -> ()  [unwired: 5 in, 2 out]
          n231 = call "Xn.vi"("Position"=w462, "_Controller in"=w470) -> ("_Controller out"=w469:refnum<class "_Controller.lvclass">)  [unwired: 8 in, 1 out]
          n232 = local read "Testing"() -> (w465:bool)
          n233 = local read "ABORT"() -> (w467:bool)
          n234 = control-ref of="ABORT"() -> (w459:refnum<vi>)
          n235 = call "WAIT 0.vi"("reference"=w459, "_Controller in"=w469) -> ("_Controller out"=w460:refnum<class "_Controller.lvclass">)  [unwired: 7 in, 2 out]
          n236 = Not(x=w467) -> (.not. x?=w466:bool)
          n237 = And(x=w465, y=w466) -> (x .and. y?=w464:bool)
          "Correction loop" <- w468
        }
      }
      frame "Terminate" {
        n238 = control-ref of="ABORT"() -> (w473:refnum<vi>)
        n239 = control-ref of="ABORT"() -> (w474:refnum<vi>)
        n240 = Unbundle(w483) -> ("queue out"=w482:refnum<queue>, "queue out"=w481:refnum<queue>, "queue out"=w480:refnum<queue>)
        n241 = case shown="False" FALSE {
          tunnel: w478 -> [w496 w513]
          tunnel: [w495 w510] -> w475
          frame False {
            n242 = call "Motor speed settings.vi"("reference (in)"=w496, "HSPD"=22000, "LSPD"=1000, "ACC"=500) -> ("reference (out)"=w501:refnum<class "_Controller.lvclass">)  [unwired: 10 in, 1 out]
            n243 = Negate(x=600 ("Position")) -> (-x=w502:i32)
            n244 = call "Xn.vi"("Position"=w502, "_Controller in"=w501) -> ("_Controller out"=w503:refnum<class "_Controller.lvclass">)  [unwired: 8 in, 1 out]
            n245 = control-ref of="ABORT"() -> (w494:refnum<vi>)
            n246 = call "WAIT 0.vi"("reference"=w494, "_Controller in"=w503) -> ("_Controller out"=w495:refnum<class "_Controller.lvclass">)  [unwired: 7 in, 2 out]
          }
          frame True {
            n247 = call "Motor speed settings.vi"("reference (in)"=w513, "HSPD"=22000, "LSPD"=1000, "ACC"=500) -> ("reference (out)"=w507:refnum<class "_Controller.lvclass">)  [unwired: 10 in, 1 out]
            n248 = Negate(x=80000 ("Position")) -> (-x=w508:i32)
            n249 = call "Xn.vi"("Position"=w508, "_Controller in"=w507) -> ("_Controller out"=w511:refnum<class "_Controller.lvclass">)  [unwired: 8 in, 1 out]
            n250 = control-ref of="ABORT"() -> (w512:refnum<vi>)
            n251 = call "WAIT 0.vi"("reference"=w512, "_Controller in"=w511) -> ("_Controller out"=w510:refnum<class "_Controller.lvclass">)  [unwired: 7 in, 2 out]
          }
        }
        n252 = call "WAIT 0.vi"("reference"=w473, "_Controller in"=w476) -> ("_Controller out"=w486:refnum<class "_Controller.lvclass">)  [unwired: 7 in, 2 out]
        n253 = call "WAIT 0.vi"("reference"=w474, "_Controller in"=w477) -> ("_Controller out"=w491:refnum<class "_Controller.lvclass">)  [unwired: 7 in, 2 out]
        n254 = Release Queue(queue=w479) -> ()  [unwired: 2 in, 3 out]
        n255 = Release Queue(queue=w480) -> ()  [unwired: 2 in, 3 out]
        n256 = call <instrlib>:"send_receive_command.vi"("reference (in)"=w486, "ASCII Command (in)"="SR0=1") -> ("reference (out)"=w487:refnum<class "_Controller.lvclass">)  [unwired: 13 in, 4 out]
        n257 = Release Queue(queue=w481) -> ()  [unwired: 2 in, 3 out]
        n258 = call <instrlib>:"send_receive_command.vi"("reference (in)"=w491, "ASCII Command (in)"="SR0=1") -> ("reference (out)"=w490:refnum<class "_Controller.lvclass">)  [unwired: 13 in, 4 out]
        n259 = Release Queue(queue=w482) -> ()  [unwired: 2 in, 3 out]
        n260 = call <instrlib>:"close_connection.vi"("reference (in)"=w487) -> ()  [unwired: 17 in, 2 out]
        n261 = call <instrlib>:"close_connection.vi"("reference (in)"=w490) -> ()  [unwired: 17 in, 2 out]
        n262 = call <instrlib>:"send_receive_command.vi"("reference (in)"=w475, "ASCII Command (in)"="SR0=1") -> ("reference (out)"=w492:refnum<class "_Controller.lvclass">)  [unwired: 13 in, 4 out]
        n263 = call <instrlib>:"close_connection.vi"("reference (in)"=w492) -> ("error out"=w472:errorcluster)  [unwired: 17 in, 1 out]
        n264 = local read "ABORT"() -> (w485:bool)
        n265 = case shown="False" w485 {
          tunnel: [w514 w515] -> w484
          tunnel: w472 -> [_ _]
          frame False {
            w514 = TRUE ("Value (Signaling)")
            n266 = property on="ABORT" class="Bool (strict)"("Val(Sgnl)"=w514) -> ()  [unwired: 2 in, 2 out]
            n267 = local write "Completed"(w514) -> ()
          }
          frame True {
            w515 = TRUE ("Value (Signaling)")
            n268 = local write "Aborted"(w515) -> ()
          }
        }
      }
    }
  }
  n269 = Format Into String(Queue_names."x-axis ref queue" ("Enum")) -> (resulting string=w17:string)  [unwired: 3 in, 1 out]
  n270 = Format Into String(Queue_names."y-axis ref queue" ("Enum")) -> (resulting string=w18:string)  [unwired: 3 in, 1 out]
  n271 = Format Into String(Queue_names."z-axis ref queue" ("Enum")) -> (resulting string=w16:string)  [unwired: 3 in, 1 out]
  n272 = Obtain Queue(name (unnamed)=w16, element data type=w2) -> (queue out=w8:refnum<queue>, error out=w7:errorcluster)  [unwired: 3 in, 1 out]
  n273 = Obtain Queue(name (unnamed)=w17, element data type=w2) -> (queue out=w10:refnum<queue>, error out=w9:errorcluster)  [unwired: 3 in, 1 out]
  n274 = Obtain Queue(name (unnamed)=w18, element data type=w2) -> (queue out=w12:refnum<queue>, error out=w11:errorcluster)  [unwired: 3 in, 1 out]
  n275 = while "Manual Control Enabling Loop" {
    tunnel: w12 -> [w531]
    tunnel: w11 -> [w530]
    tunnel: w10 -> [w529]
    tunnel: w9 -> [w528]
    tunnel: w8 -> [w527]
    tunnel: w7 -> [w526]
    tunnel: [w521] -> w6
    tunnel: [w520] -> w5
    tunnel: [w519] -> w4
    stop <- w532 stop-if-true
    n276 = Preview Queue Element(queue=w527, error in (no error)=w526) -> (queue out=w525:refnum<queue>, element=w518:refnum<class "_Controller.lvclass">)  [unwired: 1 in, 2 out]
    n277 = Preview Queue Element(queue=w529, error in (no error)=w528) -> (queue out=w524:refnum<queue>, element=w517:refnum<class "_Controller.lvclass">)  [unwired: 1 in, 2 out]
    n278 = Preview Queue Element(queue=w531, error in (no error)=w530) -> (queue out=w523:refnum<queue>, element=w516:refnum<class "_Controller.lvclass">)  [unwired: 1 in, 2 out]
    n279 = Bundle("queue out"=w525, "queue out"=w524, "queue out"=w523) -> (w522:T11)  [unwired: 1 in]
    n280 = event shown="[4] \"Left\": Value Change" {
      selector: _ -> [_ _ _ _ _ _ _ _ _ _]
      dyn-events: _ -> [_ _ _ _ _ _ _ _ _ _]
      timeout: _ -> [_ _ _ _ _ _ _ _ _ _]
      tunnel: w518 -> [_ _ w571 w582 _ _ _ _ _ _]
      tunnel: w517 -> [_ _ _ _ w593 w604 _ _ _ _]
      tunnel: w516 -> [_ _ _ _ _ _ w615 w626 _ _]
      tunnel: [_ _ _ _ _ _ _ _ _ w641] -> w532
      event Timeout {
        n281 = event-data() -> ()  [unwired: 1 in, 3 out]
      }
      event Key Down; Key Up {
        n282 = event-data() -> ("Type"=w534:T13, "ScanCode"=w535:i16)  [unwired: 1 in, 2 out]
        n283 = property on="Manual control" class="Bool (strict)"() -> ("Value"=w533:bool)  [unwired: 2 in, 2 out]
        n284 = case shown="True" w533 {
          tunnel: w535 -> [_ w537]
          tunnel: w534 -> [_ w536]
          frame False {
          }
          frame True {
            n285 = case shown="20" w537 {
              tunnel: w536 -> [_ w539 w544 w549 w554 w559 w564 w568]
              frame 0, Default {
              }
              frame 72 {
                # "Up"
                n286 = local read "Down"() -> (w538:bool)
                n287 = case shown="False" w538 {
                  tunnel: w539 -> [w540 _]
                  frame False {
                    n288 = case shown="\"Key Down\"" w540 {
                      frame "Null", Default {
                      }
                      frame "Key Down" {
                        n289 = property on="Up" class="Bool (strict)"("Val(Sgnl)"=TRUE) -> ()  [unwired: 2 in, 2 out]
                      }
                      frame "Key Up" {
                        n290 = property on="Up" class="Bool (strict)"("Val(Sgnl)"=FALSE) -> ()  [unwired: 2 in, 2 out]
                      }
                    }
                  }
                  frame True {
                  }
                }
              }
              frame 80 {
                # "Down"
                n291 = local read "Up"() -> (w543:bool)
                n292 = case shown="False" w543 {
                  tunnel: w544 -> [w545 _]
                  frame False {
                    n293 = case shown="\"Key Up\"" w545 {
                      frame "Null", Default {
                      }
                      frame "Key Down" {
                        n294 = property on="Down" class="Bool (strict)"("Val(Sgnl)"=TRUE) -> ()  [unwired: 2 in, 2 out]
                      }
                      frame "Key Up" {
                        n295 = property on="Down" class="Bool (strict)"("Val(Sgnl)"=FALSE) -> ()  [unwired: 2 in, 2 out]
                      }
                    }
                  }
                  frame True {
                  }
                }
              }
              frame 75 {
                # "Left"
                n296 = local read "Right"() -> (w548:bool)
                n297 = case shown="False" w548 {
                  tunnel: w549 -> [w550 _]
                  frame False {
                    n298 = case shown="\"Key Up\"" w550 {
                      frame "Null", Default {
                      }
                      frame "Key Down" {
                        n299 = property on="Left" class="Bool (strict)"("Val(Sgnl)"=TRUE) -> ()  [unwired: 2 in, 2 out]
                      }
                      frame "Key Up" {
                        n300 = property on="Left" class="Bool (strict)"("Val(Sgnl)"=FALSE) -> ()  [unwired: 2 in, 2 out]
                      }
                    }
                  }
                  frame True {
                  }
                }
              }
              frame 77 {
                # "Right"
                n301 = local read "Left"() -> (w553:bool)
                n302 = case shown="False" w553 {
                  tunnel: w554 -> [w555 _]
                  frame False {
                    n303 = case shown="\"Key Up\"" w555 {
                      frame "Null", Default {
                      }
                      frame "Key Down" {
                        n304 = property on="Right" class="Bool (strict)"("Val(Sgnl)"=TRUE) -> ()  [unwired: 2 in, 2 out]
                      }
                      frame "Key Up" {
                        n305 = property on="Right" class="Bool (strict)"("Val(Sgnl)"=FALSE) -> ()  [unwired: 2 in, 2 out]
                      }
                    }
                  }
                  frame True {
                  }
                }
              }
              frame 24 {
                # "Out"
                n306 = local read "In"() -> (w558:bool)
                n307 = case shown="False" w558 {
                  tunnel: w559 -> [w560 _]
                  frame False {
                    n308 = case shown="\"Key Up\"" w560 {
                      frame "Null", Default {
                      }
                      frame "Key Down" {
                        n309 = property on="Out" class="Bool (strict)"("Val(Sgnl)"=TRUE) -> ()  [unwired: 2 in, 2 out]
                      }
                      frame "Key Up" {
                        n310 = property on="Out" class="Bool (strict)"("Val(Sgnl)"=FALSE) -> ()  [unwired: 2 in, 2 out]
                      }
                    }
                  }
                  frame True {
                  }
                }
              }
              frame 23 {
                # "In"
                n311 = local read "Out"() -> (w563:bool)
                n312 = case shown="False" w563 {
                  tunnel: w564 -> [w565 _]
                  frame False {
                    n313 = case shown="\"Key Up\"" w565 {
                      frame "Null", Default {
                      }
                      frame "Key Down" {
                        n314 = property on="In" class="Bool (strict)"("Val(Sgnl)"=TRUE) -> ()  [unwired: 2 in, 2 out]
                      }
                      frame "Key Up" {
                        n315 = property on="In" class="Bool (strict)"("Val(Sgnl)"=FALSE) -> ()  [unwired: 2 in, 2 out]
                      }
                    }
                  }
                  frame True {
                  }
                }
              }
              frame 20 {
                n316 = case shown="\"Key Down\"" w568 {
                  frame "Null", Default {
                  }
                  frame "Key Down" {
                    n317 = local write "TARE"(TRUE ("TARE")) -> ()
                  }
                }
              }
            }
          }
        }
      }
      event "Up": Value Change {
        n318 = event-data() -> ()  [unwired: 1 in, 1 out]
        n319 = property on="Manual control" class="Bool (strict)"() -> ("Value"=w570:bool)  [unwired: 2 in, 2 out]
        n320 = case shown="True" w570 {
          tunnel: w571 -> [_ w572]
          frame False {
          }
          frame True {
            n321 = local read "Up"() -> (w573:bool)
            n322 = case shown="True" w573 {
              tunnel: w572 -> [w577 w580]
              frame False {
                n323 = call <instrlib>:"send_receive_command.vi"("reference (in)"=w577, "ASCII Command (in)"="STOP") -> ("reference (out)"=w575:refnum<class "_Controller.lvclass">)  [unwired: 13 in, 4 out]
                n324 = property on="Down" class="Bool (strict)"("DisabledEnum"=T6."Enabled" ("Disabled")) -> ()  [unwired: 2 in, 2 out]
                n325 = call "WAITX.vi"("_Controller in"=w575) -> ()  [unwired: 8 in, 3 out]
              }
              frame True {
                n326 = call-dynamic "jogMotor.vi"("Controller in"=w580, "dir"=linear_direction."NEG (-)") -> ()  [unwired: 14 in, 4 out]
                n327 = property on="Down" class="Bool (strict)"("DisabledEnum"=T6."Disabled" ("Disabled")) -> ()  [unwired: 2 in, 2 out]
              }
            }
          }
        }
      }
      event "Down": Value Change {
        n328 = event-data() -> ()  [unwired: 1 in, 1 out]
        n329 = property on="Manual control" class="Bool (strict)"() -> ("Value"=w581:bool)  [unwired: 2 in, 2 out]
        n330 = case shown="True" w581 {
          tunnel: w582 -> [_ w584]
          frame False {
          }
          frame True {
            n331 = local read "Down"() -> (w583:bool)
            n332 = case shown="True" w583 {
              tunnel: w584 -> [w588 w591]
              frame False {
                n333 = call <instrlib>:"send_receive_command.vi"("reference (in)"=w588, "ASCII Command (in)"="STOP") -> ("reference (out)"=w586:refnum<class "_Controller.lvclass">)  [unwired: 13 in, 4 out]
                n334 = property on="Up" class="Bool (strict)"("DisabledEnum"=T6."Enabled" ("Disabled")) -> ()  [unwired: 2 in, 2 out]
                n335 = call "WAITX.vi"("_Controller in"=w586) -> ()  [unwired: 8 in, 3 out]
              }
              frame True {
                n336 = call-dynamic "jogMotor.vi"("Controller in"=w591, "dir"=linear_direction."POS (+)") -> ()  [unwired: 14 in, 4 out]
                n337 = property on="Up" class="Bool (strict)"("DisabledEnum"=T6."Disabled" ("Disabled")) -> ()  [unwired: 2 in, 2 out]
              }
            }
          }
        }
      }
      event "Left": Value Change {
        n338 = event-data() -> ()  [unwired: 1 in, 1 out]
        n339 = property on="Manual control" class="Bool (strict)"() -> ("Value"=w592:bool)  [unwired: 2 in, 2 out]
        n340 = case shown="True" w592 {
          tunnel: w593 -> [_ w595]
          frame False {
          }
          frame True {
            n341 = local read "Left"() -> (w594:bool)
            n342 = case shown="True" w594 {
              tunnel: w595 -> [w599 w602]
              frame False {
                n343 = call <instrlib>:"send_receive_command.vi"("reference (in)"=w599, "ASCII Command (in)"="STOP") -> ("reference (out)"=w597:refnum<class "_Controller.lvclass">)  [unwired: 13 in, 4 out]
                n344 = call "WAITX.vi"("_Controller in"=w597) -> ()  [unwired: 8 in, 3 out]
                n345 = property on="Right" class="Bool (strict)"("DisabledEnum"=T6."Enabled" ("Disabled")) -> ()  [unwired: 2 in, 2 out]
              }
              frame True {
                n346 = call-dynamic "jogMotor.vi"("Controller in"=w602, "dir"=linear_direction."NEG (-)") -> ()  [unwired: 14 in, 4 out]
                n347 = property on="Right" class="Bool (strict)"("DisabledEnum"=T6."Disabled" ("Disabled")) -> ()  [unwired: 2 in, 2 out]
              }
            }
          }
        }
      }
      event "Right": Value Change {
        n348 = event-data() -> ()  [unwired: 1 in, 1 out]
        n349 = property on="Manual control" class="Bool (strict)"() -> ("Value"=w603:bool)  [unwired: 2 in, 2 out]
        n350 = case shown="True" w603 {
          tunnel: w604 -> [_ w606]
          frame False {
          }
          frame True {
            n351 = local read "Right"() -> (w605:bool)
            n352 = case shown="False" w605 {
              tunnel: w606 -> [w610 w613]
              frame False {
                n353 = call <instrlib>:"send_receive_command.vi"("reference (in)"=w610, "ASCII Command (in)"="STOP") -> ("reference (out)"=w608:refnum<class "_Controller.lvclass">)  [unwired: 13 in, 4 out]
                n354 = call "WAITX.vi"("_Controller in"=w608) -> ()  [unwired: 8 in, 3 out]
                n355 = property on="Left" class="Bool (strict)"("DisabledEnum"=T6."Enabled" ("Disabled")) -> ()  [unwired: 2 in, 2 out]
              }
              frame True {
                n356 = call-dynamic "jogMotor.vi"("Controller in"=w613, "dir"=linear_direction."POS (+)") -> ()  [unwired: 14 in, 4 out]
                n357 = property on="Left" class="Bool (strict)"("DisabledEnum"=T6."Disabled" ("Disabled")) -> ()  [unwired: 2 in, 2 out]
              }
            }
          }
        }
      }
      event "Out": Value Change {
        n358 = event-data() -> ()  [unwired: 1 in, 1 out]
        n359 = property on="Manual control" class="Bool (strict)"() -> ("Value"=w614:bool)  [unwired: 2 in, 2 out]
        n360 = case shown="True" w614 {
          tunnel: w615 -> [_ w617]
          frame False {
          }
          frame True {
            n361 = local read "Out"() -> (w616:bool)
            n362 = case shown="True" w616 {
              tunnel: w617 -> [w621 w624]
              frame False {
                n363 = call <instrlib>:"send_receive_command.vi"("reference (in)"=w621, "ASCII Command (in)"="STOP") -> ("reference (out)"=w619:refnum<class "_Controller.lvclass">)  [unwired: 13 in, 4 out]
                n364 = property on="In" class="Bool (strict)"("DisabledEnum"=T6."Enabled" ("Disabled")) -> ()  [unwired: 2 in, 2 out]
                n365 = call "WAITX.vi"("_Controller in"=w619) -> ()  [unwired: 8 in, 3 out]
              }
              frame True {
                n366 = call-dynamic "jogMotor.vi"("Controller in"=w624, "dir"=linear_direction."NEG (-)") -> ()  [unwired: 14 in, 4 out]
                n367 = property on="In" class="Bool (strict)"("DisabledEnum"=T6."Disabled" ("Disabled")) -> ()  [unwired: 2 in, 2 out]
              }
            }
          }
        }
      }
      event "In": Value Change {
        n368 = event-data() -> ()  [unwired: 1 in, 1 out]
        n369 = property on="Manual control" class="Bool (strict)"() -> ("Value"=w625:bool)  [unwired: 2 in, 2 out]
        n370 = case shown="True" w625 {
          tunnel: w626 -> [_ w628]
          frame False {
          }
          frame True {
            n371 = local read "In"() -> (w627:bool)
            n372 = case shown="True" w627 {
              tunnel: w628 -> [w632 w633]
              frame False {
                n373 = call <instrlib>:"send_receive_command.vi"("reference (in)"=w632, "ASCII Command (in)"="STOP") -> ("reference (out)"=w630:refnum<class "_Controller.lvclass">)  [unwired: 13 in, 4 out]
                n374 = call "WAITX.vi"("_Controller in"=w630) -> ()  [unwired: 8 in, 3 out]
                n375 = property on="Out" class="Bool (strict)"("DisabledEnum"=T6."Enabled" ("Disabled")) -> ()  [unwired: 2 in, 2 out]
              }
              frame True {
                n376 = call-dynamic "jogMotor.vi"("Controller in"=w633, "dir"=linear_direction."POS (+)") -> ()  [unwired: 14 in, 4 out]
                n377 = property on="Out" class="Bool (strict)"("DisabledEnum"=T6."Disabled" ("Disabled")) -> ()  [unwired: 2 in, 2 out]
              }
            }
          }
        }
      }
      event "Approach": Value Change {
        n378 = event-data() -> ()  [unwired: 1 in, 1 out]
        n379 = local read "Manual control"() -> (w636:bool)
        n380 = case shown="True" w636 {
          frame False {
          }
          frame True {
            n381 = local read "Approach"() -> (w637:bool)
            n382 = case shown="False" w637 {
              frame False {
              }
              frame True {
                n383 = flat-sequence {
                  tunnel: [FALSE ("Approach")] -> w638
                  frame #0 {
                    n384 = Wait Until Next ms Multiple(millisecond multiple=u32 300) -> ()  [unwired: 1 out]
                  }
                }
                n385 = local write "Approach"(w638) -> ()
              }
            }
          }
        }
      }
      event "ABORT": Value Change {
        n386 = event-data() -> ()  [unwired: 1 in, 1 out]
        n387 = local read "ABORT"() -> (w642:bool)
        n388 = case shown="False" w642 {
          tunnel: [FALSE TRUE] -> w641
          frame False {
          }
          frame True {
          }
        }
      }
    }
    n389 = Unbundle(w522) -> ("queue out"=w521:refnum<queue>, "queue out"=w520:refnum<queue>, "queue out"=w519:refnum<queue>)
  }
  n390 = Release Queue(queue=w6) -> ()  [unwired: 2 in, 3 out]
  n391 = Release Queue(queue=w5) -> ()  [unwired: 2 in, 3 out]
  n392 = Release Queue(queue=w4) -> ()  [unwired: 2 in, 3 out]
  n393 = while "Logic Loop" {
    shift-right: [w650] -> _
    shift-left: Logic_states."Initialize" ("Enum") -> [w651]
    shift-right: [w648] -> _
    shift-left: _ -> [w647]
    shift-right: [w646] -> _
    shift-left: _ -> [w645]
    stop <- w649 stop-if-true
    n394 = case shown="\"Process\"" w651 {
      tunnel: [w656 Logic_states."Terminate" ("Enum") _] -> w650
      tunnel: [_ _ TRUE] -> w649
      tunnel: [w665 w727 _] -> w648
      tunnel: w647 -> [_ w727 w840]
      tunnel: [w653 _ _] -> w646
      tunnel: w645 -> [_ w701 _]
      frame "Initialize", Default {
        n395 = call <vilib>:"Check if File or Folder Exists.vi"("path"="Save file name") -> ("file or folder exists?"=w663:bool, "dup path"=w662:path)  [unwired: 8 in, 1 out]
        n396 = case shown="True" w663 {
          tunnel: w662 -> [w690 w693]
          tunnel: [TRUE ("T button?") w698] -> w660
          tunnel: [w690 w693] -> w661
          tunnel: [FALSE w697] -> w657
          frame False {
          }
          frame True {
            n397 = Strip Path(path=w693) -> (name=w692:string)  [unwired: 1 out]
            n398 = Concatenate Strings("Warning!\nThis File already exists: " ("message"), "\r", w692) -> (w694:string)
            n399 = Two Button Dialog(message=w694, 1:"Abort" ("F button name (\"Cancel\")"), 2:"Overwrite" ("T button name (\"OK\")")) -> (T button?=w698:bool)
            n400 = Not(x=w698) -> (.not. x?=w697:bool)
            n401 = property on="ABORT" class="Bool (strict)"("Val(Sgnl)"=w697) -> ()  [unwired: 2 in, 2 out]
          }
        }
        n402 = case shown="True" w660 {
          tunnel: w661 -> [_ w688]
          tunnel: [_ w673] -> w653
          frame False {
          }
          frame True {
            n403 = local read "Sampling frequency (rate)"() -> (w682:T1)
            n404 = local read "Track Radius (mm)"() -> (w680:T1)
            n405 = local read "Steady State COFs"() -> (w669:dbl[])
            n406 = local read "Velocity"() -> (w681:dbl)
            n407 = local read "Wear cycles"() -> (w679:i32)
            n408 = Number To Decimal String(number=w682) -> (decimal integer string=w678:string)  [unwired: 1 in]
            n409 = Number To Decimal String(number=w681) -> (decimal integer string=w677:string)  [unwired: 1 in]
            n410 = Number To Decimal String(number=w680) -> (decimal integer string=w676:string)  [unwired: 1 in]
            n411 = Number To Decimal String(number=w679) -> (decimal integer string=w675:string)  [unwired: 1 in]
            n412 = Number To Decimal String(number=w669) -> (decimal integer string=w668:string[])  [unwired: 1 in]
            n413 = Build Array (concatenate)("Sampling fequency [Hz]:", w678, "Velocity [microsteps]: ", w677, "Track radius [mm]:", w676, "Cycles:", w675, "Steady State COFs:", w668) -> (w674:string[])
            n414 = call-poly <vilib>:"Write Delimited Spreadsheet.vi"("file path (dialog if empty)"=w688, "1D data"=w674) -> ("new file path (Not A Path if cancelled)"=w687:path)  [unwired: 12 in, 1 out]
            n415 = call-poly <vilib>:"Write Delimited Spreadsheet.vi"("file path (dialog if empty)"=w687, "1D data"=string[] ["Fx", "Fy", "Fz", "Tx", "Ty", "Tz", "Angular Position"], "append to file? (new file:F)"=TRUE) -> ("new file path (Not A Path if cancelled)"=w673:path)  [unwired: 11 in, 1 out]
          }
        }
        n416 = Format Into String(Queue_names."Cell queue name" ("Enum")) -> (resulting string=w654:string)  [unwired: 3 in, 1 out]
        n417 = Obtain Queue(name (unnamed)=w654, element data type=dbl[] []) -> (queue out=w666:refnum<queue>, error out=w664:errorcluster)  [unwired: 3 in, 1 out]
        n418 = Bundle("queue out"=w666, "error out"=w664) -> (w665:T7)  [unwired: 1 in]
        n419 = Select(t=Logic_states."Terminate" ("Enum"), s=w657, f=Logic_states."Process" ("Enum")) -> (s? t:f=w656:T5)
      }
      frame "Process" {
        n420 = Unbundle(w727) -> ("queue out"=w704:refnum<queue>, "error out"=w703:errorcluster)
        n421 = local read "Sampling frequency (rate)"() -> (w724:T1)
        n422 = while "Saving Data" {
          tunnel: w701 -> [w824]
          tunnel: w704 -> [w823]
          tunnel: w703 -> [w822]
          stop <- w830 stop-if-true
          w827 = u16 2 items=["x-load", "y-load", "z-load", "x-torque", "y-torque", "z-torque"]
          n423 = Flush Queue(queue=w823, error in (no error)=w822) -> (remaining elements=w828:cluster{dbl[]}[])  [unwired: 2 out]
          n424 = for {
            tunnel: w828 -> [w833] mode=indexing
            tunnel: [w832] -> w826 mode=indexing
            n425 = Unbundle(w833) -> (w832:dbl[])
          }
          n426 = call-poly <vilib>:"Write Delimited Spreadsheet.vi"("file path (dialog if empty)"=w824, "2D data"=w826, "append to file? (new file:F)"=TRUE) -> ()  [unwired: 11 in, 2 out]
          n427 = Index Array(array=w826, index (col)=w827) -> (element=w825:dbl[])  [unwired: 1 in]
          n428 = Negate(x=w825) -> (-x=→"Dequeued Data":dbl[])
          n429 = local read "ABORT"() -> (w830:bool)
        }
        n430 = Less Or Equal?(x=w724, y=u16 50) -> (x <= y?=w726:bool)
        n431 = Reciprocal(x=w724) -> (1/x=w723:dbl)
        n432 = Multiply(x=1000.0, y=w723) -> (x*y=w721:dbl)
        n433 = Format Into String(Queue_names."Feedback" ("Enum")) -> (resulting string=w707:string)  [unwired: 3 in, 1 out]
        n434 = Select(t=w721, s=w726, f=10.0) -> (s? t:f=w712:dbl)
        n435 = Divide(x=w712, y=1000.0) -> (x/y=w713:dbl)
        n436 = Obtain Queue(max queue size (-1, unlimited)=1, name (unnamed)=w707, element data type=0) -> (queue out=w706:refnum<queue>)  [unwired: 2 in, 2 out]
        n437 = Format Into String(Queue_names."to PID" ("Enum")) -> (resulting string=w717:string)  [unwired: 3 in, 1 out]
        n438 = Obtain Queue(max queue size (-1, unlimited)=1, name (unnamed)=w717, element data type=0.0) -> (queue out=w714:refnum<queue>)  [unwired: 2 in, 2 out]
        n439 = while "Averaging" {
          tunnel: w712 -> [w783]
          tunnel: w714 -> [w768]
          tunnel: [w758] -> w702
          tunnel: w701 -> [w753]
          stop <- w785 stop-if-true
          w766 = u16 5 items=["x-load", "y-load", "z-load", "x-torque", "y-torque", "z-torque"]
          w782 = u16 5 items=["x-load", "y-load", "z-load", "x-torque", "y-torque", "z-torque"]
          w788 = u16 2 items=["x-load", "y-load", "z-load", "x-torque", "y-torque", "z-torque"]
          n440 = local read "Number of Previous Points"() -> (w757:i32)
          n441 = local read "Current reading"() -> (w761:dbl[])
          n442 = Wait (ms)(milliseconds to wait=w783) -> ()  [unwired: 1 out]
          n443 = local read "Track Radius (mm)"() -> (w763:T1)
          n444 = Index Array(array=w761, index=w766) -> (element=→"Torque":dbl)
          n445 = Index Array(array=w761, index=w788) -> (element=w789:dbl)
          n446 = Index Array(array=w761, index=w782) -> (element=w764:dbl)
          n447 = Negate(x=w789) -> (-x=w786:dbl)
          n448 = local read "Averaging Level"() -> (w784:i32)
          n449 = Divide(x=w764, y=w763) -> (x/y=w762:dbl)
          n450 = control-ref of="Mean z"() -> (w787:refnum<vi>)
          n451 = local read "Averaging Level"() -> (w780:i32)
          n452 = control-ref of="Mean Force from Torque"() -> (w781:refnum<vi>)
          n453 = call "Smoothing.vi"("Averaging Level"=w784, "Input reading"=w786, "Array in"=w787) -> ("mean"=w767:dbl)  [unwired: 8 in]
          "Smooth z" <- w767
          "Actual Load" <- w767
          n454 = call "Smoothing.vi"("Averaging Level"=w780, "Input reading"=w762, "Array in"=w781) -> ("mean"=w779:dbl)  [unwired: 8 in]
          "Smooth Force from Torque" <- w779
          n455 = local read "Testing Load [N]"() -> (w778:dbl)
          n456 = local read "Manual control"() -> (w775:bool)
          n457 = local read "ABORT"() -> (w769:bool)
          n458 = Divide(x=w779, y=w767) -> (x/y=w759:dbl)
          "Estimated friction coefficient" <- w759
          n459 = Greater Or Equal?(x=w767, y=w778) -> (x >= y?=w777:bool)
          n460 = Not(x=w775) -> (.not. x?=w774:bool)
          n461 = And(x=w777, y=w774) -> (x .and. y?=w776:bool)
          n462 = Greater?(x=w767, y=33.0) -> (0:w772:bool)
          n463 = Or(x=w776, y=w769) -> (x .or. y?=w770:bool)
          n464 = local read "Number of Previous Points"() -> (w760:i32)
          n465 = control-ref of="Mean Estimated Friction Coefficient"() -> (w751:refnum<vi>)
          n466 = local read "Steady State COFs"() -> (w750:dbl[])
          n467 = call "Smoothing.vi"("Averaging Level"=w760, "Input reading"=w759, "Array in"=w751) -> ("mean"=w752:dbl)  [unwired: 8 in]
          n468 = And(x=w772, y=w774) -> (x .and. y?=w771:bool)
          n469 = Build Array (concatenate)(w750, w752) -> (w754:dbl[])
          n470 = Array Size(array=w754) -> (size(s)=w756:i32)
          n471 = Greater?(x=w756, y=w757) -> (0:w755:bool)
          n472 = case shown="True" w755 {
            tunnel: w754 -> [_ w791]
            tunnel: w753 -> [_ w790]
            frame False {
            }
            frame True {
              n473 = while {
                tunnel: w790 -> [w798]
                tunnel: w791 -> [w794]
                stop <- w793 stop-if-true
                n474 = local read "Number of Previous Points"() -> (w800:i32)
                n475 = Array Size(array=w794) -> (size(s)=w805:i32)
                n476 = Decrement(x=w805) -> (x-1=w804:i32)
                n477 = Subtract(x=w804, y=w800) -> (x-y=w803:i32)
                n478 = Array Size(array=w794) -> (size(s)=w809:i32)
                n479 = Decrement(x=w809) -> (x-1=w808:i32)
                n480 = Array Subset(array=w794, index=w803, length=w800) -> (w802:dbl[])
                n481 = Index Array(array=w794, index=w808) -> (element=w795:dbl)
                n482 = local read "Maximum COF Difference"() -> (w810:i32)
                n483 = Add Array Elements(numeric array=w802) -> (sum=w801:dbl)
                n484 = Divide(x=w801, y=w800) -> (x/y=w799:dbl)
                n485 = Subtract(x=w795, y=w799) -> (x-y=w807:dbl)
                n486 = Absolute Value(x=w807) -> (abs(x)=w806:dbl)
                n487 = Greater Or Equal?(x=w806, y=w810) -> (x >= y?=w796:bool)
                n488 = while {
                  shift-right: [w812] -> _
                  shift-left: dbl[] [] -> [w814]
                  tunnel: w796 -> [w815]
                  tunnel: w795 -> [w813]
                  tunnel: [w812] -> w792
                  stop <- w811 stop-if-true
                  n489 = case shown="False" w815 {
                    tunnel: w814 -> [w816 w819]
                    tunnel: w813 -> [_ w818]
                    tunnel: [w816 w817] -> w812
                    frame False {
                    }
                    frame True {
                      n490 = Build Array (concatenate)(w819, w818) -> (w817:dbl[])
                    }
                  }
                  n491 = local read "ABORT"() -> (w811:bool)
                }
                n492 = call-poly <vilib>:"Write Delimited Spreadsheet.vi"("file path (dialog if empty)"=w798, "1D data"=w792) -> ()  [unwired: 12 in, 2 out]
                n493 = local read "ABORT"() -> (w793:bool)
                n494 = local write "Steady State COFs"(w792) -> ()
              }
            }
          }
          n495 = case shown="False" w770 {
            frame False {
            }
            frame True {
              n496 = local write "Approaching"(FALSE ("Approaching")) -> ()
            }
          }
          n497 = Lossy Enqueue Element(queue=w768, element=w767) -> (queue out=w758:refnum<queue>)  [unwired: 1 in, 3 out]
          n498 = case shown="False" w771 {
            frame False {
            }
            frame True {
              n499 = property on="ABORT" class="Bool (strict)"("Val(Sgnl)"=TRUE ("Value (Signaling)")) -> ()  [unwired: 2 in, 2 out]
            }
          }
          n500 = local read "ABORT"() -> (w785:bool)
        }
        n501 = while "PID" {
          tunnel: w713 -> [w734]
          tunnel: w714 -> [w731]
          tunnel: w706 -> [w730]
          tunnel: [w729] -> w705
          i -> [w732]
          stop <- w733 stop-if-true
          n502 = local read "Testing"() -> (w728:bool)
          n503 = case shown="True" w728 {
            tunnel: w734 -> [_ _]
            tunnel: w731 -> [_ w748]
            tunnel: w730 -> [w736 w744]
            tunnel: [w736 w743] -> w729
            frame False {
              n504 = Wait (ms)(milliseconds to wait=u32 250) -> ()  [unwired: 1 out]
            }
            frame True {
              n505 = Dequeue Element(queue=w748) -> (element=w740:dbl, error out=w745:errorcluster)  [unwired: 2 in, 2 out]
              n506 = call <vilib>:"Clear Errors.vi"("error in (no error)"=w745) -> ()  [unwired: 5 in, 2 out]
              n507 = local read "Testing Load [N]"() -> (w741:dbl)
              n508 = call-poly <vilib>:"PID.vi"("output range"="output range", "PID gains"="PID gains", "process variable"=w740, "setpoint"=w741) -> ("dt out (s)"=→"dt out (s)":dbl, "output"=w747:dbl)  [unwired: 6 in]
              "Correction [N]" <- w747
              n509 = Quotient & Remainder(x=w747, y=0.015) -> (floor(x/y)=w739:dbl)  [unwired: 1 out]
              "correction [p]" <- w739
              n510 = To Long Integer(number=w739) -> (32bit integer=w742:i32)
              n511 = Lossy Enqueue Element(queue=w744, element=w742) -> (queue out=w743:refnum<queue>)  [unwired: 1 in, 3 out]
            }
          }
          n512 = local read "ABORT"() -> (w733:bool)
          "to PID" <- w732
        }
        n513 = Release Queue(queue=w705) -> ()  [unwired: 2 in, 3 out]
        n514 = Release Queue(queue=w702) -> ()  [unwired: 2 in, 3 out]
      }
      frame "Terminate" {
        n515 = Initialize Array(0.0 ("element")) -> (w836:dbl[])  [unwired: 1 in]
        n516 = Initialize Array(0.0 ("element")) -> (w837:dbl[])  [unwired: 1 in]
        n517 = Unbundle(w840) -> ("queue out"=w839:refnum<queue>, "error out"=w838:errorcluster)
        n518 = local write "Mean Force from Torque"(w837) -> ()
        n519 = local write "Mean z"(w836) -> ()
        n520 = Release Queue(queue=w839, error in (no error)=w838) -> ()  [unwired: 1 in, 3 out]
      }
    }
  }
  "x-position" <- 0 ("x-position")
  "Angular Position" <- 0.0 ("Angular Position")
